vi "Failure.vi"(1 "TestFailure In":refnum<class "TestFailure.lvclass">) -> (0 "Failure":errorcluster)   [LabVIEW 2019, in "TestFailure.lvclass"]
uses:
  TestFailure.lvclass
  TestFailure.lvclass/TestFailure.ctl
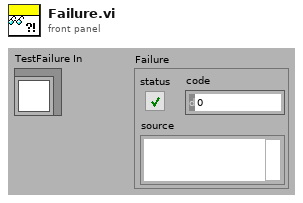
[diagram p1: front panel]
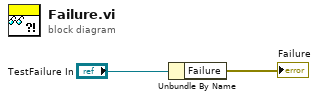
[diagram p0: block diagram]
diagram:
  n1 = Unbundle By Name("TestFailure In") -> ("Failure"=→"Failure":errorcluster)
